vi "sub_calculate-covariance.vi"(9 "pw":T1, 10 "px":T1, 11 "x_est":T1) -> (3 "cov out":T1)   [LabVIEW 2019]
uses:
  <vilib>/Analysis/Matrix/Datatypes/RealMatrix.ctl
  <vilib>/Analysis/baseanly.llb/Real A x B.vi
  <vilib>/Analysis/Matrix/Numeric/Subtract/Subtract - RM,RM.vi
  <vilib>/Analysis/Matrix/Numeric/Multiply/Multiply - RM,R.vi
  <vilib>/Analysis/Matrix/Numeric/Add/Add - RM,RM.vi
  <vilib>/Analysis/Matrix/Numeric/Subtract/Subtract (Elementwise) - R,RM.vi
  <vilib>/Analysis/Matrix/NI_Matrix.lvlib
  <vilib>/Analysis/NI_AALBase.lvlib
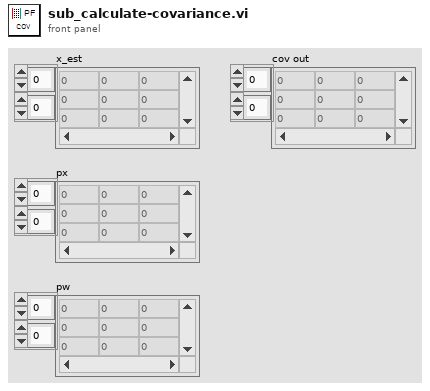
[diagram p1: front panel]
types:
  T1 = typedef "NI_Matrix.lvlib/RealMatrix.ctl" = dbl[][]
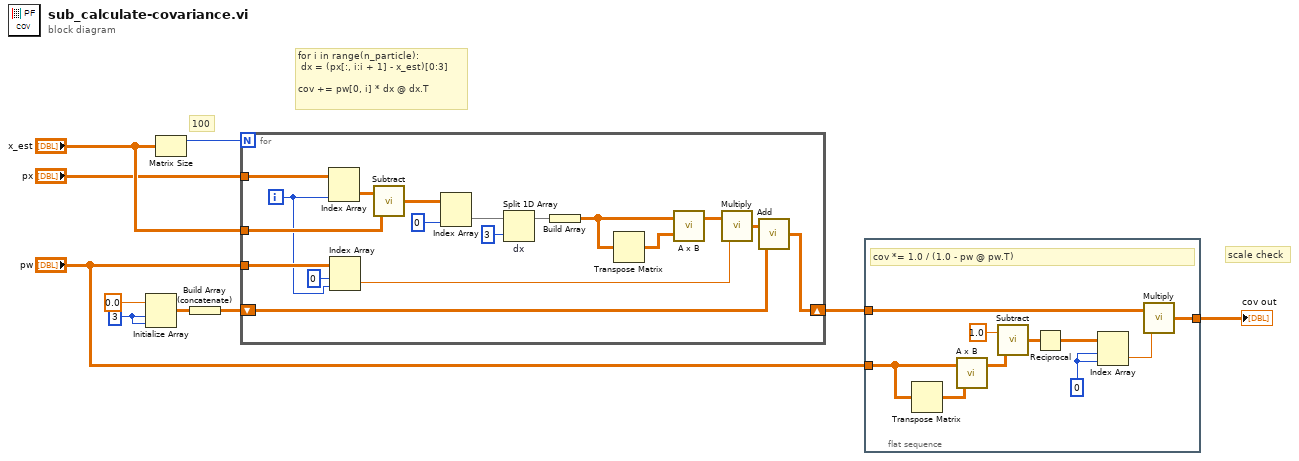
[diagram p0: block diagram]
diagram:
  w2 = 3 ("dimension size")
  # "scale check"
  # "for i in range(n_particle):\n\tdx = (px[:, i:i + 1] - x_est)[0:3]\n        \ncov += pw[0, i] * dx @ dx.T"
  # "100"
  n1 = Initialize Array(0.0 ("element"), w2, w2) -> (w4:dbl[][])
  n2 = Matrix Size(0:"x_est") -> (1:w3:i32)  [unwired: 1 out]
  n3 = Build Array (concatenate)(w4) -> (w7:T1)
  n4 = for {
    N: w3 -> [_]
    shift-right: [w15] -> w9
    shift-left: w7 -> [w16]
    tunnel: "px" -> [w28]
    tunnel: "x_est" -> [w27]
    tunnel: "pw" -> [w23]
    i -> [w21]
    n5 = Index Array(array=w28, index (col)=w21) -> (element=w14:T1)  [unwired: 1 in]
    n6 = Index Array(array=w23, index (row)=0, index (col)=w21) -> (element=w19:dbl)
    n7 = call-poly <vilib>:"Subtract.vi"("Real Matrix B"=w27, "Real Matrix A"=w14) -> ("A - B"=w26:T1)
    n8 = Index Array(array=w26, index (col)=0 ("index (row)")) -> (element=w25:dbl[])  [unwired: 1 in]
    n9 = Split 1D Array "dx"(array=w25, index=3) -> (first subarray=w20:dbl[])  [unwired: 1 out]
    n10 = Build Array(w20) -> (w12:T1)
    n11 = Transpose Matrix(1:w12) -> (0:w11:T1)
    n12 = call-poly <vilib>:"A x B.vi"("B"=w11, "A"=w12) -> ("A x B"=w18:T1)  [unwired: 1 out]
    n13 = call-poly <vilib>:"Multiply.vi"("Real Scalar c"=w19, "Real Matrix A"=w18) -> ("A * c"=w17:T1)
    n14 = call-poly <vilib>:"Add.vi"("Real Matrix B"=w16, "Real Matrix A"=w17) -> ("A + B"=w15:T1)
  }
  n15 = flat-sequence {
    tunnel: "pw" -> [w37]
    tunnel: w9 -> [w30]
    tunnel: [w29] -> w10
    frame #0 {
      w32 = 0 ("index (row)")
      # "cov *= 1.0 / (1.0 - pw @ pw.T)"
      n16 = Transpose Matrix(1:w37) -> (0:w38:T1)
      n17 = call-poly <vilib>:"A x B.vi"("B"=w38, "A"=w37) -> ("A x B"=w36:T1)  [unwired: 1 out]
      n18 = call-poly <vilib>:"Subtract.vi"("Real Matrix A"=w36, "Real Scalar c"=1.0) -> ("c - A"=w34:T1)
      n19 = Reciprocal(x=w34) -> (1/x=w33:T1)
      n20 = Index Array(array=w33, index (row)=w32, index (col)=w32) -> (element=w31:dbl)
      n21 = call-poly <vilib>:"Multiply.vi"("Real Scalar c"=w31, "Real Matrix A"=w30) -> ("A * c"=w29:T1)
    }
  }
  "cov out" <- w10
